vi "setDeviceName.vi"(8 "error in":errorcluster, 10 "device name in":string, 11 "connection ID":refnum<k5>) -> (0 "error out":errorcluster, 3 "connection ID out":refnum<k5>)   [LabVIEW 2019]
panel:
  in  "Set Command":string="com.attocube.system.setDeviceName"
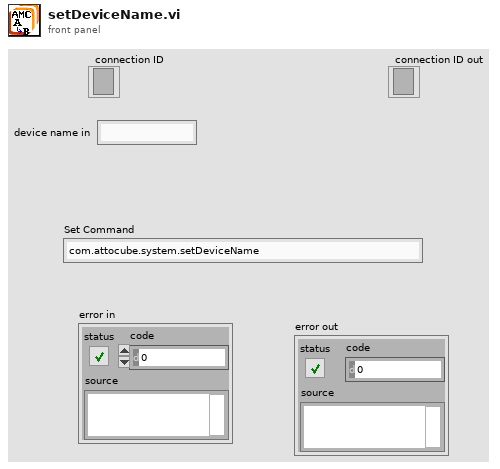
[diagram p1: front panel]
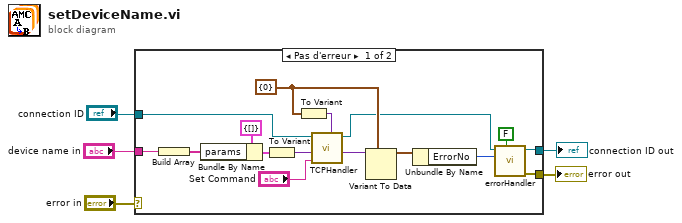
[diagram p0: block diagram]
diagram:
  n1 = case shown="Pas d'erreur" "error in" {
    selector: "error in" -> [_ w23]
    tunnel: [w20 w23] -> w5
    tunnel: "device name in" -> [w21 _]
    tunnel: "connection ID" -> [w18 w22]
    tunnel: [w19 w22] -> w2
    frame No Error {
      w9 = cluster{"ErrorNo":i64} {"ErrorNo"=0} ("input cluster")
      n2 = Build Array(w21) -> (w6:string[])
      n3 = Bundle By Name(cluster=cluster{"params":string[]} {"params"=[]} ("input cluster"), "params"=w6) -> (w14:cluster{"params":string[]})
      n4 = To Variant(anything=w14) -> (Variant=w15:variant)
      n5 = To Variant(anything=w9) -> (Variant=w10:variant)
      n6 = call "TCPHandler.vi"("result Types"=w10, "method"="Set Command", "params"=w15, "connection ID"=w18) -> ("result"=w12:variant, "connection ID"=w7:refnum<k5>)  [unwired: 5 in, 1 out]
      n7 = Variant To Data(type=w9, Variant=w12) -> (data=w16:cluster{"ErrorNo":i64})  [unwired: 1 in, 1 out]
      n8 = Unbundle By Name(w16) -> ("ErrorNo"=w17:i64)
      n9 = call "errorHandler.vi"("show popup"=FALSE, "error number"=w17, "connection ID"=w7) -> ("error out"=w20:errorcluster, "connection ID"=w19:refnum<k5>)  [unwired: 7 in]
    }
    frame Error {
    }
  }
  "error out" <- w5
  "connection ID out" <- w2
